vi "Get Producer Values.vi"(8 "error in":errorcluster, 11 "Power Supply Cluster.lvclass":refnum<class "Power Supply Cluster.lvclass">) -> (0 "error out":errorcluster, 1 "Producer Ch":T1(array[cluster]), 2 "Producer Control":T2, 3 "Power Supply Cluster.lvclass out":refnum<class "Power Supply Cluster.lvclass">)   [LabVIEW 2023, in "Power Supply Cluster.lvclass"]
uses:
  Power Supply Cluster.lvclass
  Power Supply Cluster.lvclass/Power Supply Cluster.ctl
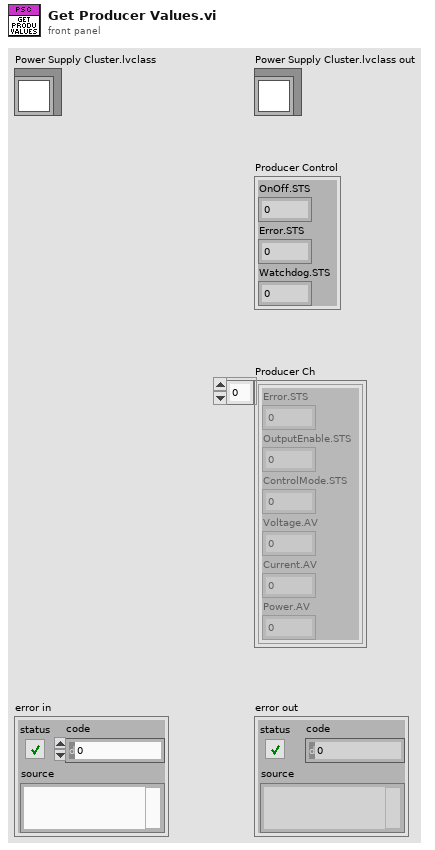
[diagram p1: front panel]
types:
  T1 = cluster{"Error.STS":i32, "OutputEnable.STS":i32, "ControlMode.STS":u16, "Voltage.AV":dbl, "Current.AV":dbl, "Power.AV":dbl}[]
  T2 = cluster{"OnOff.STS":i32, "Error.STS":i32, "Watchdog.STS":i32}
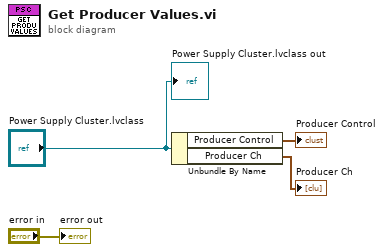
[diagram p0: block diagram]
diagram:
  n1 = Unbundle By Name("Power Supply Cluster.lvclass") -> ("Producer Control"=→"Producer Control":T2, "Producer Ch"=→"Producer Ch":T1)
  "Power Supply Cluster.lvclass out" <- "Power Supply Cluster.lvclass"
  "error out" <- "error in"
